vi "Write Default to File.vi"(8 "error in (no error)":errorcluster, 9 "Name":string, 10 "Path":path, 11 "ObjectSettings in":refnum<class "ObjectSettings.lvclass">) -> (0 "error out":errorcluster, 3 "ObjectSettings out":refnum<class "ObjectSettings.lvclass">)   [LabVIEW 2019, in "ObjectSettings.lvclass"]
uses:
  ObjectSettings.lvclass
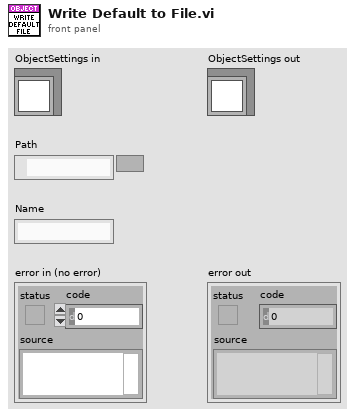
[diagram p1: front panel]
types:
  T1 = typedef "ObjectSettings.lvclass/DefaultCluster.ctl" = cluster{"Enabled":bool, "Direction":u16, "Speed":cluster{"Schedule":u16, "Settings":cluster{"KVPs":cluster{"Key":string, "Value":string}[]}}, "Voltage":cluster{"Schedule":u16, "Settings":cluster{"KVPs":cluster{"Key":string, "Value":string}[]}}, "Resistance":enum16{"Open", "Discharge Tip", "0 ohm", "100 kohm", "10 Mohm", "1 Gohm"}}
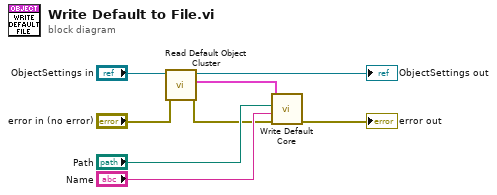
[diagram p0: block diagram]
diagram:
  n1 = call "Read Default Object Cluster.vi"("error in (no error)"="error in (no error)", "ObjectSettings in"="ObjectSettings in") -> ("error out"=w3:errorcluster, "Default Object"=w1:T1, "ObjectSettings out"=→"ObjectSettings out":refnum<class "ObjectSettings.lvclass">)  [unwired: 7 in]
  n2 = call "Write Default Core.vi"("error in (no error)"=w3, "Name"="Name", "Path"="Path", "Cluster In"=w1) -> ("error out"=→"error out":errorcluster)  [unwired: 6 in, 1 out]
